vi "WriteStatusFlag.vi"(8 "error in (no error)":errorcluster, 10 "Message Status":T1 items=["Simple", "Dialog", "PVUpdate", "Dialog + PVUpdate", "N/A"], 11 "CS++Message in":refnum<class "CS++Message.lvclass">) -> (0 "error out":errorcluster, 3 "CS++Message out":refnum<class "CS++Message.lvclass">)   [LabVIEW 2015, in "CS++Message.lvlib" / "CS++Message.lvclass"]
uses:
  CS++Message.lvclass
  MessageStatus.ctl
  CS++Message.lvclass/CS++Message.ctl
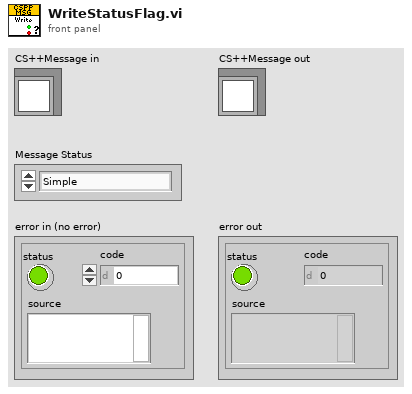
[diagram p1: front panel]
types:
  T1 = typedef "CS++Message.lvlib/CS++Message.lvclass/MessageStatus.ctl" = u16
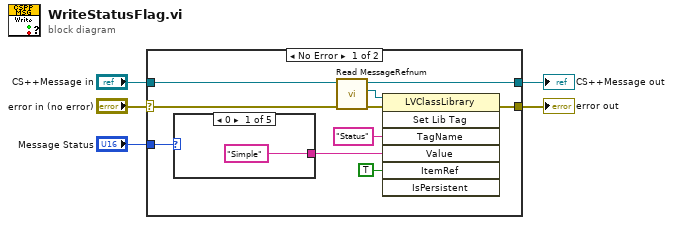
[diagram p0: block diagram]
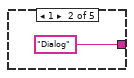
[diagram p2: hidden frame]
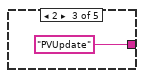
[diagram p3: hidden frame]
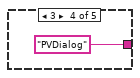
[diagram p4: hidden frame]
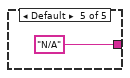
[diagram p5: hidden frame]
diagram:
  n1 = case shown="No Error" "error in (no error)" {
    selector: "error in (no error)" -> [w13 w22]
    tunnel: [w10 w22] -> w4
    tunnel: [w14 w21] -> w2
    tunnel: "CS++Message in" -> [w15 w21]
    tunnel: "Message Status" -> [w8 _]
    frame No Error {
      n2 = case shown="0" w8 {
        tunnel: ["Simple" ("Tag Name") "Dialog" ("Tag Name") "PVUpdate" ("Tag Name") "PVDialog" ("Tag Name") "N/A" ("Tag Name")] -> w7
        frame 0 {
        }
        frame 1 {
        }
        frame 2 {
        }
        frame 3 {
        }
        frame Default {
        }
      }
      n3 = call "Read MessageRefnum.vi"("error in (no error)"=w13, "CS++Message in"=w15) -> ("error out"=w11:errorcluster, "MessageRefnum"=w12:refnum<vi>, "CS++Message out"=w14:refnum<class "CS++Message.lvclass">)  [unwired: 7 in]
      n4 = invoke class="LVClassLibrary" method="Set Lib Tag"(reference=w12, error in=w11, "TagName"="Status" ("Tag Name"), "Value"=w7, "ItemRef"=TRUE ("Is Persistent")) -> (error out=w10:errorcluster)  [unwired: 2 in, 6 out]
    }
    frame Error {
    }
  }
  "error out" <- w4
  "CS++Message out" <- w2
